vi "Interpolation2.vi"(1 "Normalize to # of Data Points":dbl, 2 "Original Array":dbl[](array[numeric])) -> (0 "Normalized Array":dbl[](array[numeric]))   [LabVIEW 2011]
panel:
  out "new scan rate":dbl format="%.2f"
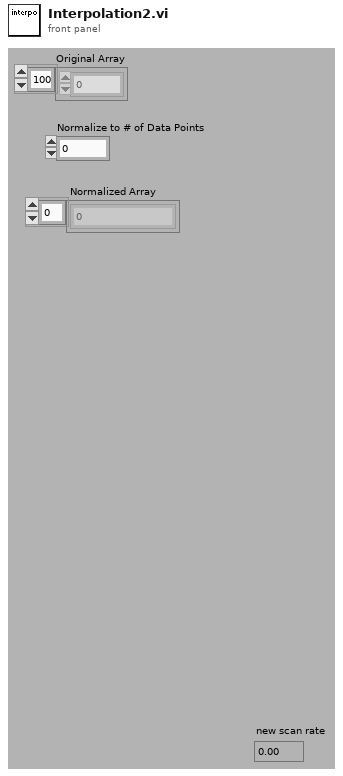
[diagram p1: front panel]
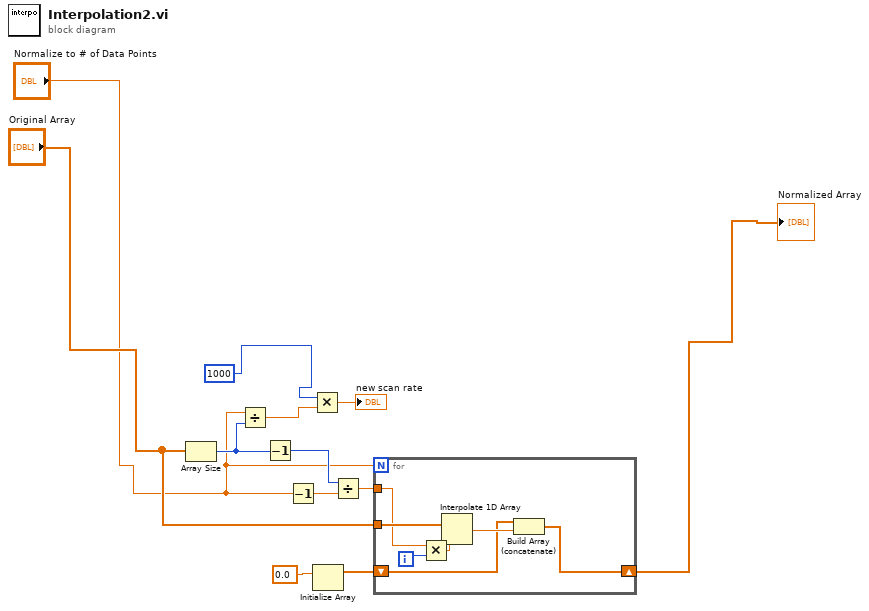
[diagram p0: block diagram]
diagram:
  n1 = Array Size(array="Original Array") -> (size(s)=w10:i32)
  n2 = Divide(x="Normalize to # of Data Points", y=w10) -> (x/y=w8:dbl)
  n3 = Decrement(x=w10) -> (x-1=w5:i32)
  n4 = Decrement(x="Normalize to # of Data Points") -> (x-1=w6:dbl)
  n5 = Multiply(x=1000, y=w8) -> (x*y=→"new scan rate":dbl)
  n6 = Initialize Array(sgl 0.0) -> (w12:sgl[])  [unwired: 1 in]
  n7 = Divide(x=w5, y=w6) -> (x/y=w7:dbl)
  n8 = for {
    N: "Normalize to # of Data Points" -> [_]
    tunnel: "Original Array" -> [w17]
    tunnel: w7 -> [w16]
    shift-right: [w13] -> w1
    shift-left: w12 -> [w14]
    i -> [w18]
    n9 = Multiply(x=w16, y=w18) -> (x*y=w15:dbl)
    n10 = Interpolate 1D Array(1:w15, 2:w17) -> (0:w19:dbl)
    n11 = Build Array (concatenate)(w14, w19) -> (w13:dbl[])
  }
  "Normalized Array" <- w1
